vi "Write Project Path.vi"(8 "error in (no error)":errorcluster, 10 "Project Path":string, 11 "EXE Build in":refnum<class "LabVIEW Build.lvclass">) -> (0 "error out":errorcluster, 3 "EXE Build out":refnum<class "LabVIEW Build.lvclass">)   [LabVIEW 2014, in "LabVIEW Build.lvclass"]
uses:
  LabVIEW Build.lvclass
  LabVIEW Build.lvclass/LabVIEW Build.ctl
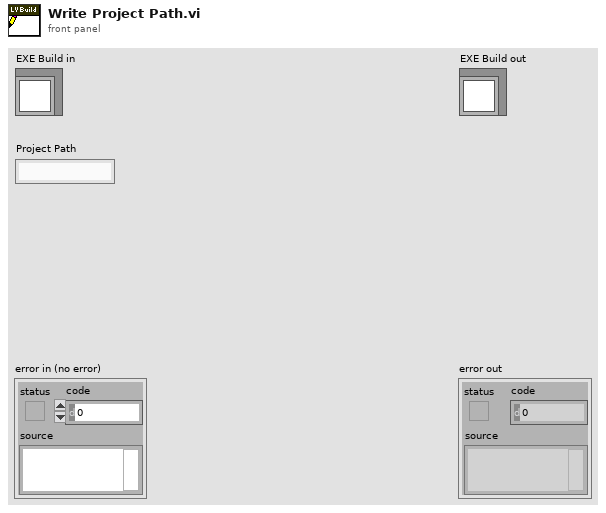
[diagram p1: front panel]
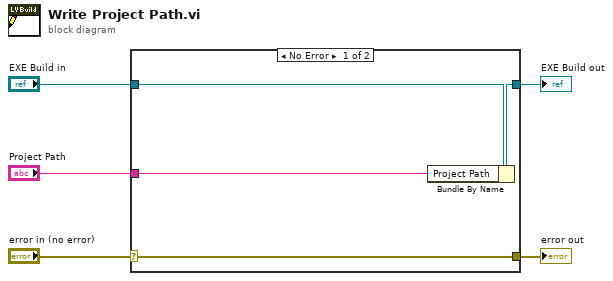
[diagram p0: block diagram]
diagram:
  n1 = case shown="No Error" "error in (no error)" {
    selector: "error in (no error)" -> [w9 w10]
    tunnel: [w9 w10] -> w4
    tunnel: [w7 w11] -> w2
    tunnel: "EXE Build in" -> [w8 w11]
    tunnel: "Project Path" -> [w6 _]
    frame No Error {
      n2 = Bundle By Name(cluster=w8, "Project Path"=w6) -> (w7:refnum<class "LabVIEW Build.lvclass">)
    }
    frame Error {
    }
  }
  "error out" <- w4
  "EXE Build out" <- w2
